vi "FTW-Logger-Launch.vi"(5 "FTW Logger Configuration":T2="{\n  \"Identity\": \"EventLog\",\n  \"InboxAddress\": \"lvq://127.0.0.1:*\",\n  \"PublisherAddress\": \"\",\n  \"LoggerAddress\": \"\",\n  \"EnableInboxLogging\": false,\n  \"EnableJobLogging\": false,\n  \"ApplicationName\": \"Featherweight Application\",\n  \"LoggerDirectory\": \"[UserAppData]\\\\[ApplicationName]\",\n  \"LoggerDiskThrashDelay\": 200,\n  \"DebugShowPanel\": true\n}", 11 "error in":errorcluster) -> (4 "FTW Logger Connector":refnum<class "FTW-Logger.lvclass">, 6 "Logger Address":T1, 15 "error out":errorcluster)   [LabVIEW 2012, in "FTW-Actor.lvlib" / "FTW-Logger.lvclass"]
doc: "This method launches a Logger Process which is then referred to based on its LoggerID. Normally in a LabVIEW application, an object's methods would adhere to dataflow with the object wired to the method; however, the Logger Process object likely needs to be accessed by many different portions of your application, and for this reason, it is called by reference, where the LoggerID string refers to the logger.\n\nThis method should be called as one of the very first actions in your application to reasonably ensure the buffer of logged events does not overflow. Events that are logged prior to launching the Logger Process with this method are queued, and will be logged once this process begins."
uses:
  FTW-Logger.lvclass
  Utility/FTW-Actor-Configuration.ctl
  Utility/FTW-Actor-Address.ctl
  Connector/FTW-ActorConnector.lvclass
  FTW-Actor.lvlib
panel:
  # "Inputs"
  # "Outputs"
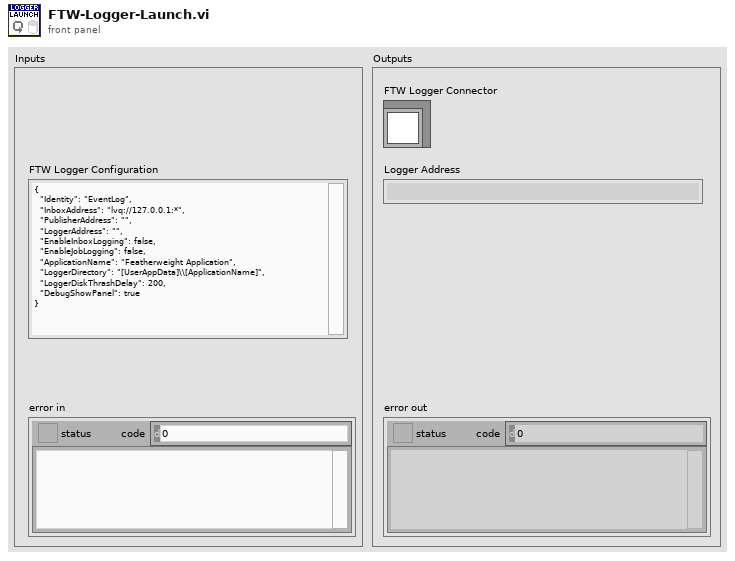
[diagram p1: front panel]
types:
  T1 = typedef "FTW-Actor.lvlib/FTW-Actor-Address.ctl" = string
  T2 = typedef "FTW-Actor.lvlib/FTW-Actor-Configuration.ctl" = string
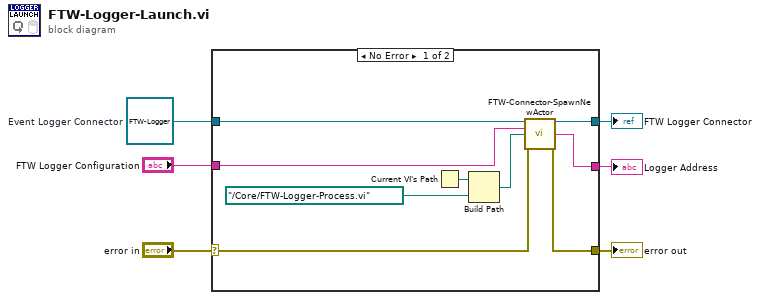
[diagram p0: block diagram]
diagram:
  w3 = refnum<class "FTW-Logger.lvclass"> refnum  # Event Logger Connector
  n1 = case shown="No Error" "error in" {
    selector: "error in" -> [w12 w17]
    tunnel: [w8 w17] -> w6
    tunnel: [w9 w16] -> w4
    tunnel: w3 -> [w13 w16]
    tunnel: "FTW Logger Configuration" -> [w10 _]
    tunnel: [w7 _] -> w1
    frame No Error {
      n2 = Current VI's Path() -> (path=w14:path)
      n3 = Build Path(base path=w14, name or relative path=path "../Core/FTW-Logger-Process.vi") -> (appended path=w11:path)
      n4 = call "FTW-Connector-SpawnNewActor.vi"("FTW Actor Connector Type"=w13, "Configuration"=w10, "Actor VI Filepath"=w11, "error in"=w12) -> ("FTW Actor Connector"=w9:refnum<class "FTW-Logger.lvclass">, "Instance Inbox Address"=w7:T1, "error out"=w8:errorcluster)  [unwired: 7 in, 2 out]
    }
    frame Error {
    }
  }
  "error out" <- w6
  "FTW Logger Connector" <- w4
  "Logger Address" <- w1
